vi "LWXPS_PositionerAnalogTrackingVelocityParametersSet.vi"(0 "Analog input name":string, 1 "Offset":dbl, 2 "Scale":dbl, 3 "Dead Band Threshold":dbl, 4 "Order":i32, 5 "Velocity":dbl, 6 "Positioner Name":string, 7 "Acceleration":dbl, 8 "XPS Reference IN":refnum<k24>, 9 "LabVIEW error IN":errorcluster) -> (14 "XPS Reference OUT":refnum<k24>, 15 "Returned error code":i32, 18 "XPS Error String":string, 19 "LabVIEW error OUT":errorcluster)   [LabVIEW 2015]
uses:
  C:/Users/Becky/Desktop/XPS-UNIFIED/LabVIEW VIs/LabVIEW Source Code/Dll/Newport.XPS.CommandInterface.dll
  Dll/Newport.XPS.CommandInterface.dll
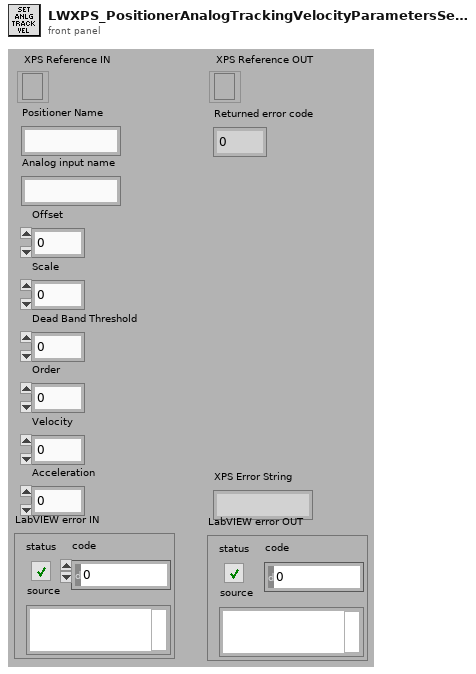
[diagram p1: front panel]
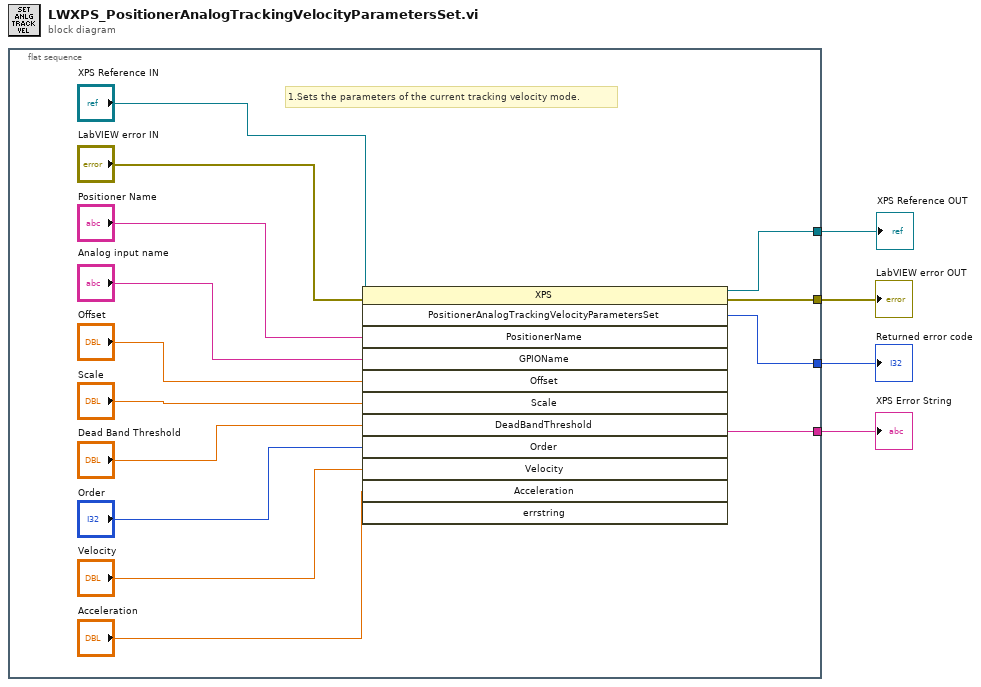
[diagram p0: block diagram]
diagram:
  n1 = flat-sequence {
    tunnel: [w10] -> w4
    tunnel: [w17] -> w3
    tunnel: [w9] -> w2
    tunnel: [w11] -> w1
    frame #0 {
      # "1.Sets the parameters of the current tracking velocity mode."
      n2 = invoke class="XPS" method="PositionerAnalogTrackingVelocityParametersSet"(reference="XPS Reference IN", error in="LabVIEW error IN", "PositionerName"="Positioner Name", "GPIOName"="Analog input name", "Offset"="Offset", "Scale"="Scale", "DeadBandThreshold"="Dead Band Threshold", "Order"="Order", "Velocity"="Velocity", "Acceleration"="Acceleration") -> (reference out=w10:refnum<k24>, error out=w17:errorcluster, "PositionerAnalogTrackingVelocityParametersSet"=w9:i32, "errstring"=w11:string)  [unwired: 2 in, 8 out]
    }
  }
  "XPS Error String" <- w1
  "XPS Reference OUT" <- w4
  "LabVIEW error OUT" <- w3
  "Returned error code" <- w2
